vi "Convert Waveform To User Defined List.vi"(7 "Waveform Shape (0: None)":i32(ring) items=["None", "Exponential", "Pulse", "Ramp", "Sine Wave", "Staircase", "Step", "Trapezoid"], 8 "error in (no error)":errorcluster {"code" format="%.0x"}, 9 "Waveform Type (1: Voltage)":i32(ring)=1 items=["Voltage"=1, "Current"=0], 10 "Channel Name (1)":string="1", 11 "VISA resource name":refnum<visa-resource-name>) -> (0 "error out":errorcluster {"code" format="%.0x"}, 3 "VISA resource name out":refnum<visa-resource-name>)   [LabVIEW 2010, in "Agilent N6700 Series.lvlib"]
doc: "This VI converts the specified waveform to a list of points in the user-defined waveform format. \n\n<b>Note:</b>\n\nWaveform capability is only available on the N6705B DC Power Analyzer."
uses:
  Agilent N6700 Series.lvlib
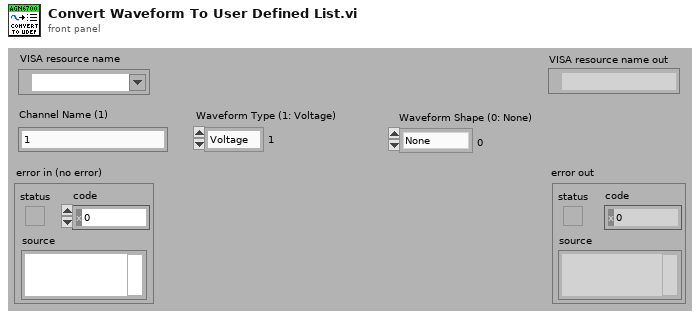
[diagram p1: front panel]
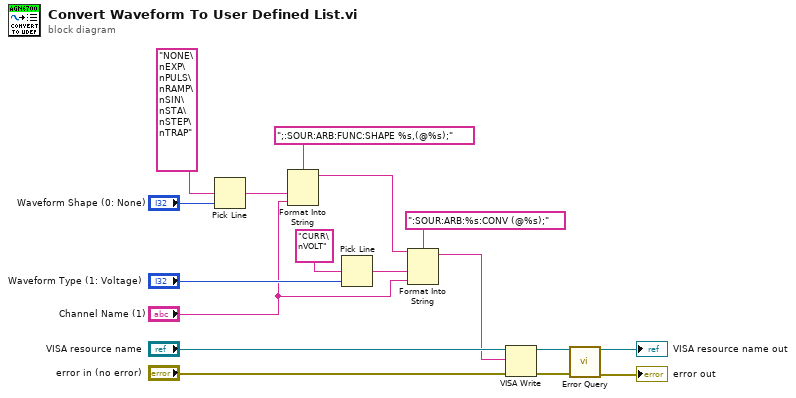
[diagram p0: block diagram]
diagram:
  n1 = Pick Line(multi-line string="NONE\nEXP\nPULS\nRAMP\nSIN\nSTA\nSTEP\nTRAP" ("string (\"\")"), line index="Waveform Shape (0: None)") -> (output string=w10:string)  [unwired: 1 in]
  n2 = Format Into String(format string=";:SOUR:ARB:FUNC:SHAPE %s,(@%s);", w10, "Channel Name (1)") -> (resulting string=w5:string)  [unwired: 2 in, 1 out]
  n3 = Pick Line(multi-line string="CURR\nVOLT" ("string (\"\")"), line index="Waveform Type (1: Voltage)") -> (output string=w7:string)  [unwired: 1 in]
  n4 = Format Into String(format string=":SOUR:ARB:%s:CONV (@%s);", initial string=w5, w7, "Channel Name (1)") -> (resulting string=w1:string)  [unwired: 1 in, 1 out]
  n5 = VISA Write(VISA resource name="VISA resource name", write buffer=w1, error in (no error)="error in (no error)") -> (VISA resource name out=w13:refnum<visa-resource-name>, error out=w12:errorcluster)  [unwired: 1 out]
  n6 = call "Error Query.vi"("VISA resource name"=w13, "error in (no error)"=w12) -> ("VISA resource name out"=→"VISA resource name out":refnum<visa-resource-name>, "error out"=→"error out":errorcluster)  [unwired: 10 in, 2 out]
